vi "Tare AP Sensor with Internal Barometer.vi"(7 "Unit ID (A)":string="A", 8 "error in":errorcluster, 11 "VISA Session In":refnum<visa-resource-name>="Alicat") -> (0 "error out":errorcluster, 3 "VISA Session Out":refnum<visa-resource-name>)   [LabVIEW 2015]
doc: "Performs a tare of the absolute presure sensor of a mass flow or absolute pressure Alicat device using the internal barometer chip. To work, the Alicat must have firmware revision 6v0 or higher and an on-board barometer chip."
uses:
  <vilib>/Instr/_visa.llb/VISA Flush IO Buffer Mask.ctl
panel:
  in  "Software Version":u8
  out "Completion text":string
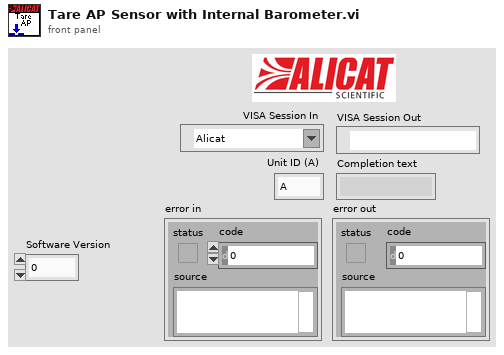
[diagram p1: front panel]
types:
  T1 = typedef "VISA Flush IO Buffer Mask.ctl" = u16
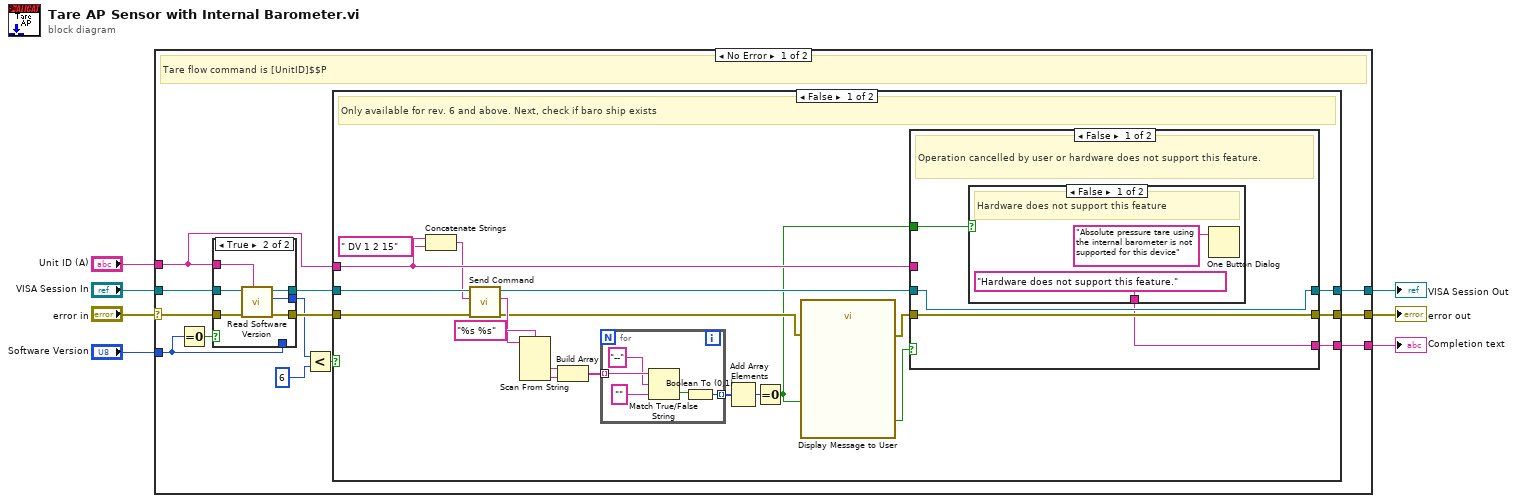
[diagram p0: block diagram]
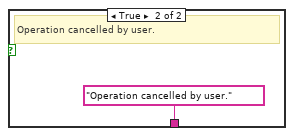
[diagram p2: hidden frame]
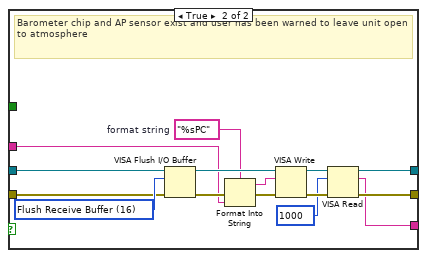
[diagram p3: hidden frame]
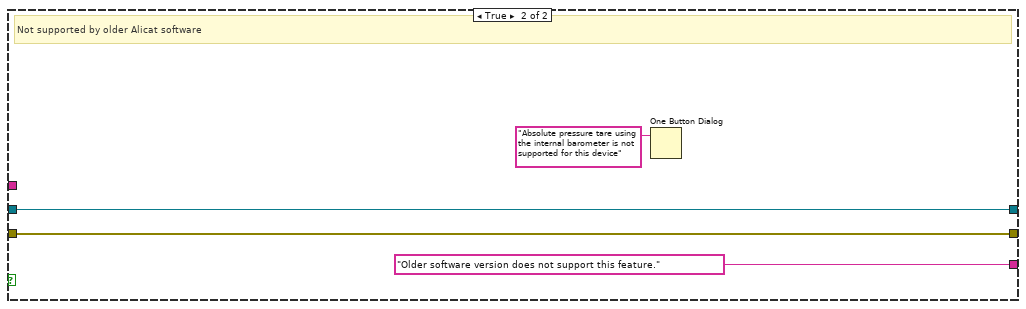
[diagram p4: hidden frame]
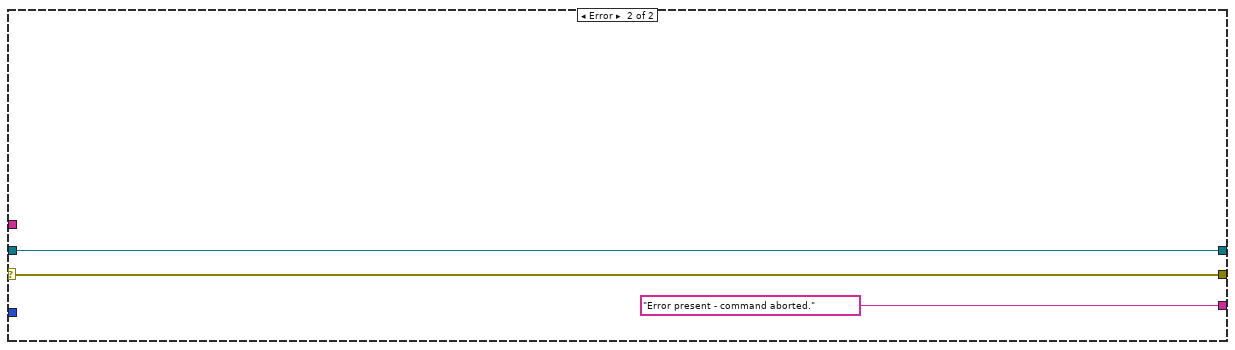
[diagram p6: hidden frame]
diagram:
  n1 = case shown="No Error" "error in" {
    selector: "error in" -> [w16 w82]
    tunnel: "VISA Session In" -> [w15 w83]
    tunnel: [w20 w83] -> w6
    tunnel: [w19 w82] -> w5
    tunnel: [w18 "Error present - command aborted." ("read buffer")] -> w3
    tunnel: "Unit ID (A)" -> [w12 _]
    tunnel: "Software Version" -> [w11 _]
    frame No Error {
      # "Tare flow command is [UnitID]$$P"
      n2 = Equal To 0?(x=w11) -> (x = 0?=w17:bool)
      n3 = case shown="True" w17 {
        tunnel: w16 -> [w73 w80]
        tunnel: w15 -> [w72 w79]
        tunnel: w12 -> [_ w78]
        tunnel: [w73 w77] -> w14
        tunnel: [w72 w76] -> w13
        tunnel: [w74 w75] -> w9
        tunnel: w11 -> [w74 _]
        frame False {
        }
        frame True {
          n4 = call "Read Software Version.vi"("Unit ID (A)"=w78, "error in"=w80, "VISA Session In"=w79) -> ("error out"=w77:errorcluster, "Software Version"=w75:u8, "VISA Session Out"=w76:refnum<visa-resource-name>)  [unwired: 6 in]
        }
      }
      n5 = Less?(x=w9, y=u8 6) -> (x < y?=w8:bool)
      n6 = case shown="False" w8 {
        tunnel: [w40 w71] -> w20
        tunnel: [w39 w70] -> w19
        tunnel: [w38 "Older software version does not support this feature." ("read buffer")] -> w18
        tunnel: w14 -> [w36 w70]
        tunnel: w13 -> [w37 w71]
        tunnel: w12 -> [w34 _]
        frame False {
          # "Only available for rev. 6 and above. Next, check if baro ship exists"
          n7 = Concatenate Strings(w34, " DV 1 2 15" ("string")) -> (w32:string)
          n8 = call "Send Command.vi"("error in"=w36, "Command"=w32, "VISA Session In"=w37) -> ("error out"=w24:errorcluster, "Response"=w25:string, "VISA Session Out"=w35:refnum<visa-resource-name>)  [unwired: 6 in]
          n9 = Scan From String(format string="%s %s", input string=w25) -> (output 1=w26:string, output 2=w27:string)  [unwired: 4 in, 3 out]
          n10 = Build Array(w26, w27) -> (w28:string[])
          n11 = for {
            tunnel: w28 -> [w45] mode=indexing
            tunnel: [w41] -> w30 mode=indexing
            n12 = Match True/False String(2:"" ("false string"), 3:"--", 4:w45) -> (0:w42:bool)  [unwired: 1 out]
            n13 = Boolean To (0,1)(Boolean=w42) -> (0, 1=w41:i16)
          }
          n14 = Add Array Elements(numeric array=w30) -> (sum=w31:i16)
          n15 = Equal To 0?(x=w31) -> (x = 0?=w21:bool)
          n16 = call "Display Message to User"("error in (no error)"=w24, "Enable"=w21) -> ("error out"=w23:errorcluster, "Continue"=w22:bool)  [unwired: 8 in]
          n17 = case shown="False" w22 {
            tunnel: w35 -> [w48 w67]
            tunnel: [w48 w66] -> w40
            tunnel: [w49 w65] -> w39
            tunnel: w34 -> [_ w55]
            tunnel: w23 -> [w49 w54]
            tunnel: [w46 w53] -> w38
            tunnel: w21 -> [w47 _]
            frame False {
              # "Operation cancelled by user or hardware does not support this feature."
              n18 = case shown="False" w47 {
                tunnel: ["Hardware does not support this feature." ("read buffer") "Operation cancelled by user." ("read buffer")] -> w46
                frame False {
                  # "Hardware does not support this feature"
                  n19 = One Button Dialog(message="Absolute pressure tare using the internal barometer is not supported for this device") -> ()  [unwired: 1 in, 1 out]
                }
                frame True {
                  # "Operation cancelled by user."
                }
              }
            }
            frame True {
              w56 = T1 16 items=["Flush Receive Buffer"=16, "Write Transmit Buffer to Device"=32, "Flush Receive Buffer (No I/O)"=64, "Flush Transmit Buffer"=128] ("Mask")
              w61 = "%sPC"  # format string
              # "Barometer chip and AP sensor exist and user has been warned to leave unit open to atmosphere"
              n20 = VISA Flush I/O Buffer(VISA resource name=w67, mask (16)=w56, error in (no error)=w54) -> (VISA resource name out=w63:refnum<visa-resource-name>, error out=w59:errorcluster)
              n21 = Format Into String(format string=w61, error in=w59, w55) -> (resulting string=w60:string, error out=w58:errorcluster)  [unwired: 1 in]
              n22 = VISA Write(VISA resource name=w63, write buffer=w60, error in (no error)=w58) -> (VISA resource name out=w62:refnum<visa-resource-name>, error out=w64:errorcluster)  [unwired: 1 out]
              n23 = VISA Read(VISA resource name=w62, byte count=u32 1000, error in (no error)=w64) -> (VISA resource name out=w66:refnum<visa-resource-name>, read buffer=w53:string, error out=w65:errorcluster)  [unwired: 1 out]
            }
          }
        }
        frame True {
          # "Not supported by older Alicat software"
          n24 = One Button Dialog(message="Absolute pressure tare using the internal barometer is not supported for this device") -> ()  [unwired: 1 in, 1 out]
        }
      }
    }
    frame Error {
    }
  }
  "error out" <- w5
  "VISA Session Out" <- w6
  "Completion text" <- w3
